vi "Is ProjectItem an lvproj, lvlib, or lvclass.vi"(8 "Error In":errorcluster, 11 "Project Item Ref":refnum<vi>) -> (0 "Error Out":errorcluster, 3 "Is the input ProjectItem reference that of an lvproj, lvlib, or lvclass?":bool)   [LabVIEW 2022 SP3]
doc: "This VI returns True if and only if the input ProjectItem Ref is that of an lvproj, lvlib or lvclass."
panel:
  out "Type String":string
  # "Development\nControls or indicators that are useful for development or testing, but which are not outputs of the VI."
  # "Input\nInputs to the VI"
  # "Output\nOutputs of the VI"
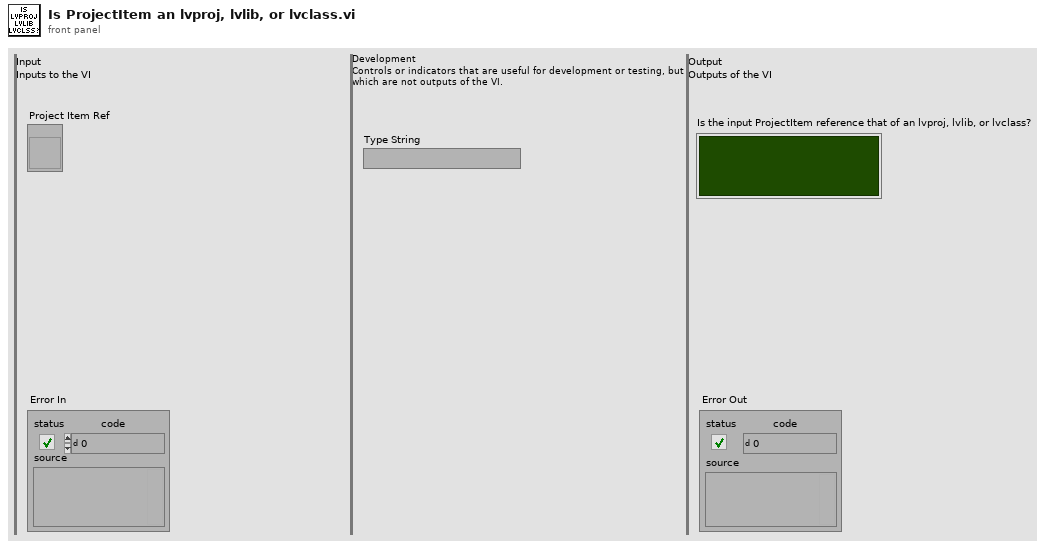
[diagram p1: front panel]
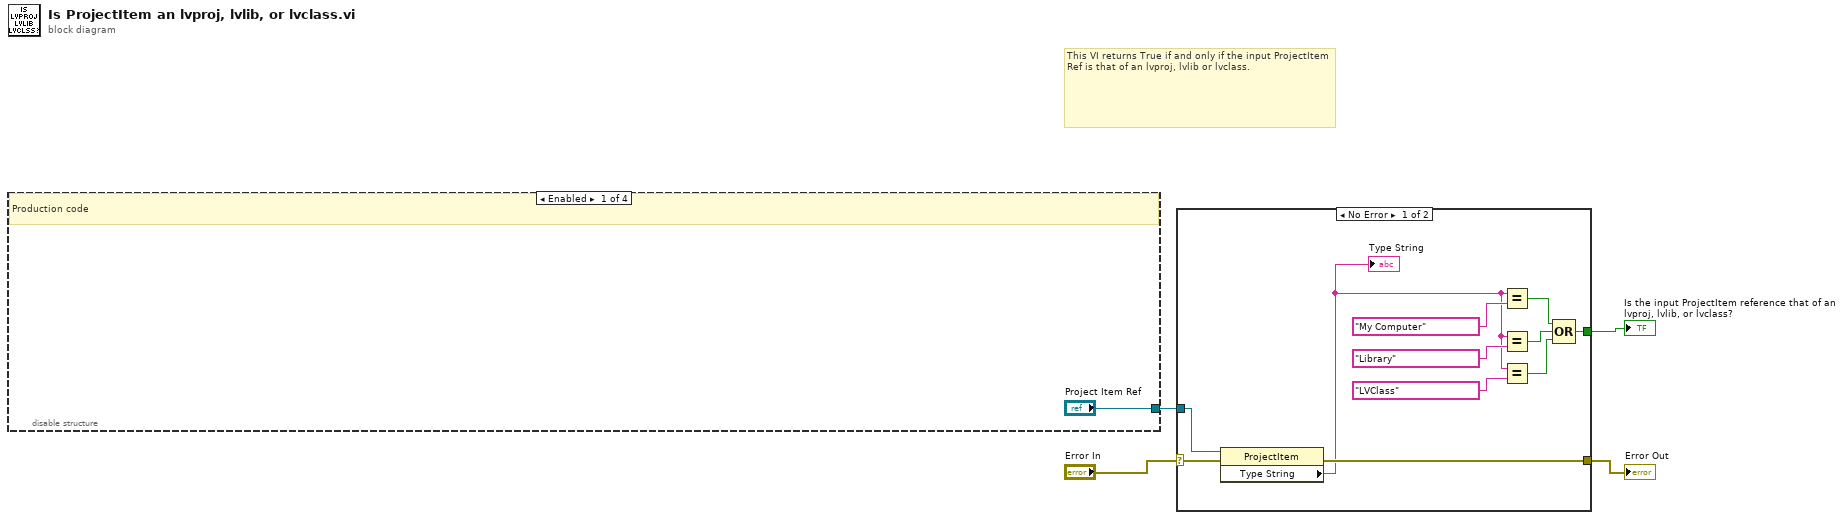
[diagram p0: block diagram]
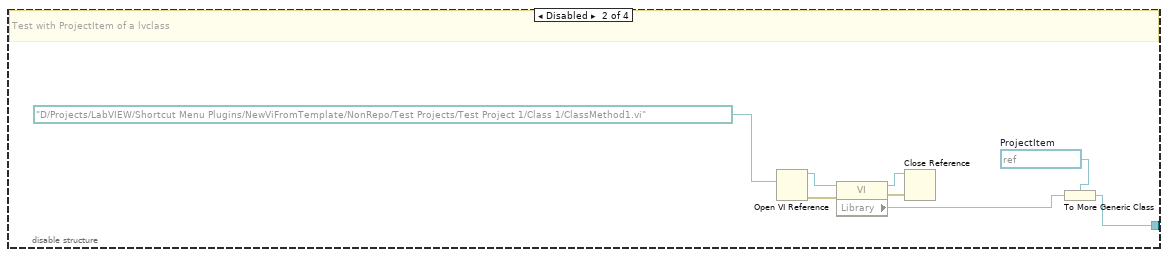
[diagram p2: hidden frame]
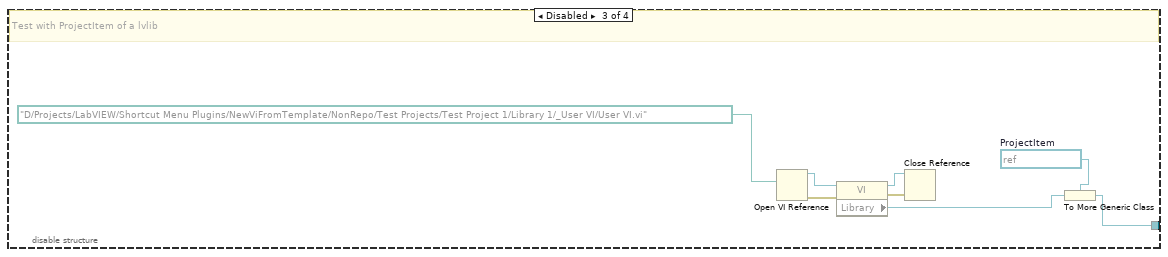
[diagram p3: hidden frame]
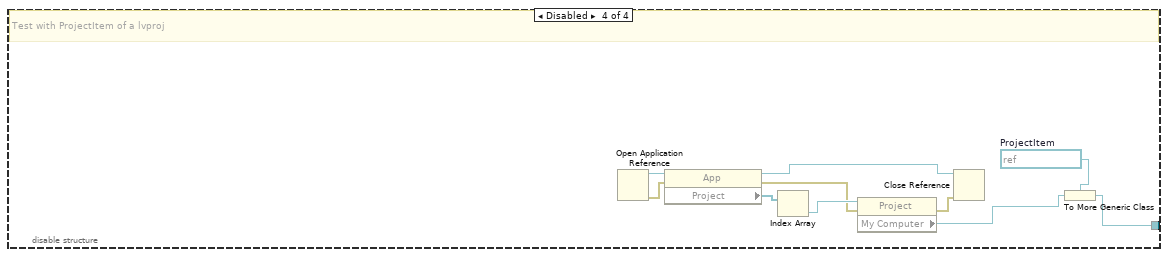
[diagram p4: hidden frame]
diagram:
  # "This VI returns True if and only if the input ProjectItem Ref is that of an lvproj, lvlib or lvclass."
  n1 = disable-structure shown="Enabled" {
    disable-tunnel: ["Project Item Ref" w9 w17 w30] -> w2
    frame Enabled {
      # "Production code"
    }
    frame Disabled {
      w10 = refnum<vi> refnum  # ProjectItem
      # "Test with ProjectItem of a lvclass"
      n2 = Open VI Reference(vi path=path "D:/Projects/LabVIEW/Shortcut Menu Plugins/NewViFromTemplate/NonRepo/Test Projects/Test Project 1/Class 1/ClassMethod1.vi") -> (vi reference=w7:refnum<vi>, error out=w12:errorcluster)  [unwired: 5 in]
      n3 = property class="VI"(reference=w7, error in=w12) -> (reference out=w6:refnum<vi>, error out=w8:errorcluster, "Library"=w11:refnum<vi>)
      n4 = Close Reference(reference=w6, error in (no error)=w8) -> ()  [unwired: 1 out]
      n5 = To More Generic Class(target class=w10, reference=w11) -> (generic class reference=w9:refnum<vi>)
    }
    frame Disabled {
      w18 = refnum<vi> refnum  # ProjectItem
      # "Test with ProjectItem of a lvlib"
      n6 = Open VI Reference(vi path=path "D:/Projects/LabVIEW/Shortcut Menu Plugins/NewViFromTemplate/NonRepo/Test Projects/Test Project 1/Library 1/_User VI/User VI.vi") -> (vi reference=w15:refnum<vi>, error out=w20:errorcluster)  [unwired: 5 in]
      n7 = property class="VI"(reference=w15, error in=w20) -> (reference out=w14:refnum<vi>, error out=w16:errorcluster, "Library"=w19:refnum<vi>)
      n8 = Close Reference(reference=w14, error in (no error)=w16) -> ()  [unwired: 1 out]
      n9 = To More Generic Class(target class=w18, reference=w19) -> (generic class reference=w17:refnum<vi>)
    }
    frame Disabled {
      w31 = refnum<vi> refnum  # ProjectItem
      # "Test with ProjectItem of a lvproj"
      n10 = Open Application Reference() -> (0:w28:errorcluster, 3:w29:refnum<vi>)  [unwired: 4 in]
      n11 = property class="App"(reference=w29, error in=w28) -> (reference out=w22:refnum<vi>, error out=w24:errorcluster, "Project"=w27:refnum<vi>[])
      n12 = Index Array(array=w27) -> (element=w26:refnum<vi>)  [unwired: 1 in]
      n13 = property class="Project"(reference=w26, error in=w24) -> (error out=w23:errorcluster, "My Computer"=w25:refnum<vi>)  [unwired: 1 out]
      n14 = Close Reference(reference=w22, error in (no error)=w23) -> ()  [unwired: 1 out]
      n15 = To More Generic Class(target class=w31, reference=w25) -> (generic class reference=w30:refnum<vi>)
    }
  }
  n16 = case shown="No Error" "Error In" {
    selector: "Error In" -> [w42 w43]
    tunnel: [w41 w43] -> w3
    tunnel: w2 -> [w40 _]
    tunnel: [w32 _] -> w1
    frame No Error {
      n17 = property class="ProjectItem"(reference=w40, error in=w42) -> (error out=w41:errorcluster, "Type String"=w34:string)  [unwired: 1 out]
      "Type String" <- w34
      n18 = Equal?(x=w34, y="My Computer") -> (x = y?=w38:bool)
      n19 = Equal?(x=w34, y="Library") -> (x = y?=w36:bool)
      n20 = Equal?(x=w34, y="LVClass") -> (x = y?=w35:bool)
      n21 = Compound Arithmetic op=OR(w38, w36, w35) -> (w32:bool)
    }
    frame Error {
    }
  }
  "Error Out" <- w3
  "Is the input ProjectItem reference that of an lvproj, lvlib, or lvclass?" <- w1
